vi "EC_Load.vi"() -> ()   [LabVIEW 2018]
uses:
  <vilib>/Utility/miscctls.llb/LVPositionTypeDef.ctl
panel:
  in  "Tab Control":enum32{"Document", "File"}(tab)
  in  "Document Path":path
  in  "Undo":bool
  in  "Document Tree":string[](tree)=["D:\\ATI_MS_InstrumentControl_08_08_15\\MSData\\Test\\Untitled.flist"]
  in  "File Tree":string[](tree)
  out "Navigate Tree:Get Path":string[](array[string])
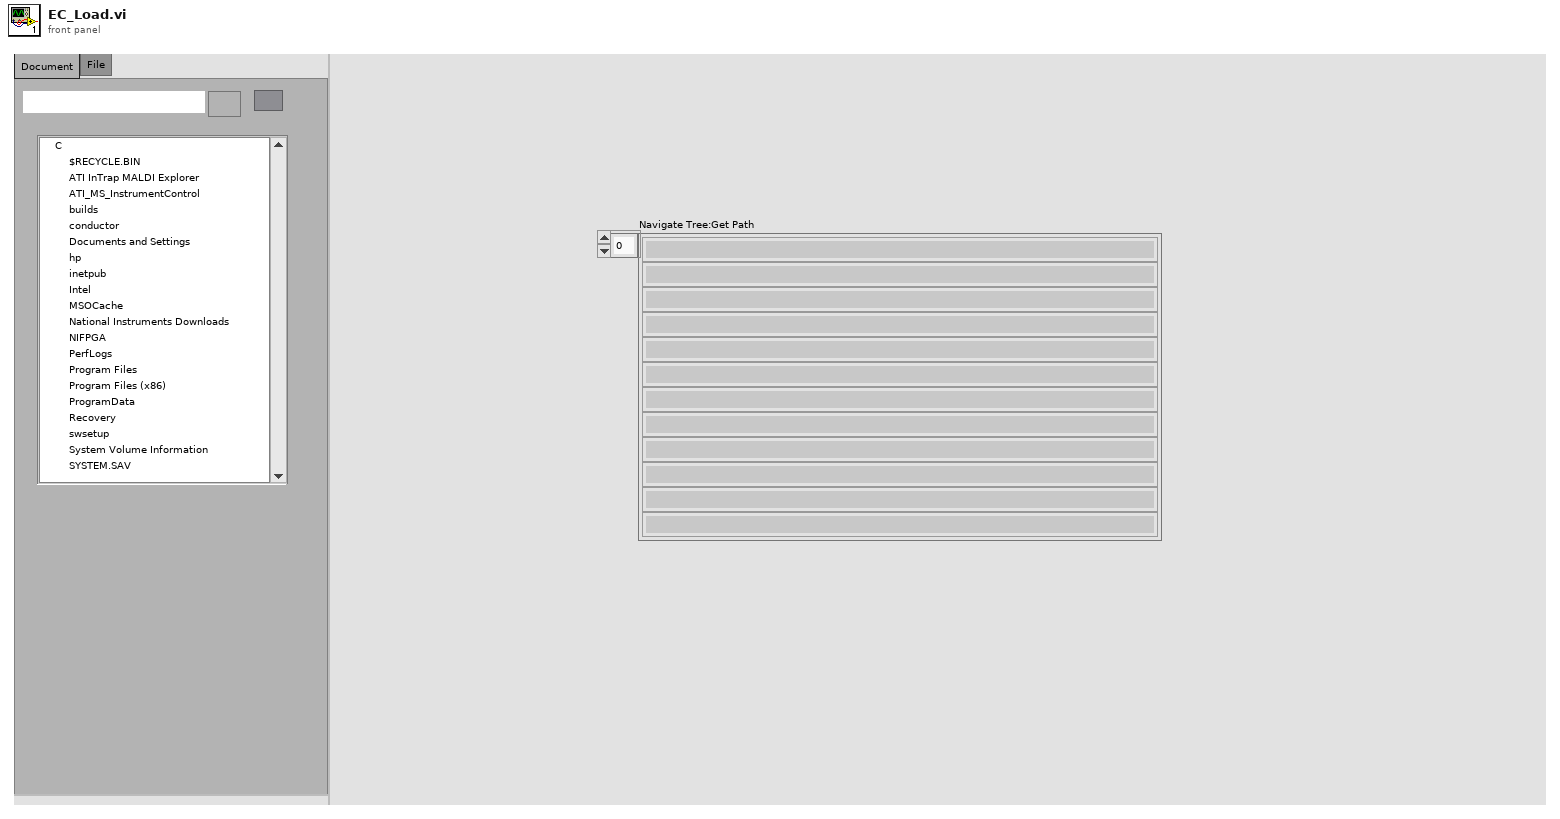
[diagram p1: front panel]
types:
  T1 = typedef "LVPositionTypeDef.ctl" = cluster{"Left":i32, "Top":i32}
  T2 = typedef "LVBoundsTypeDef.ctl" = cluster{"Width":u32, "Height":u32}
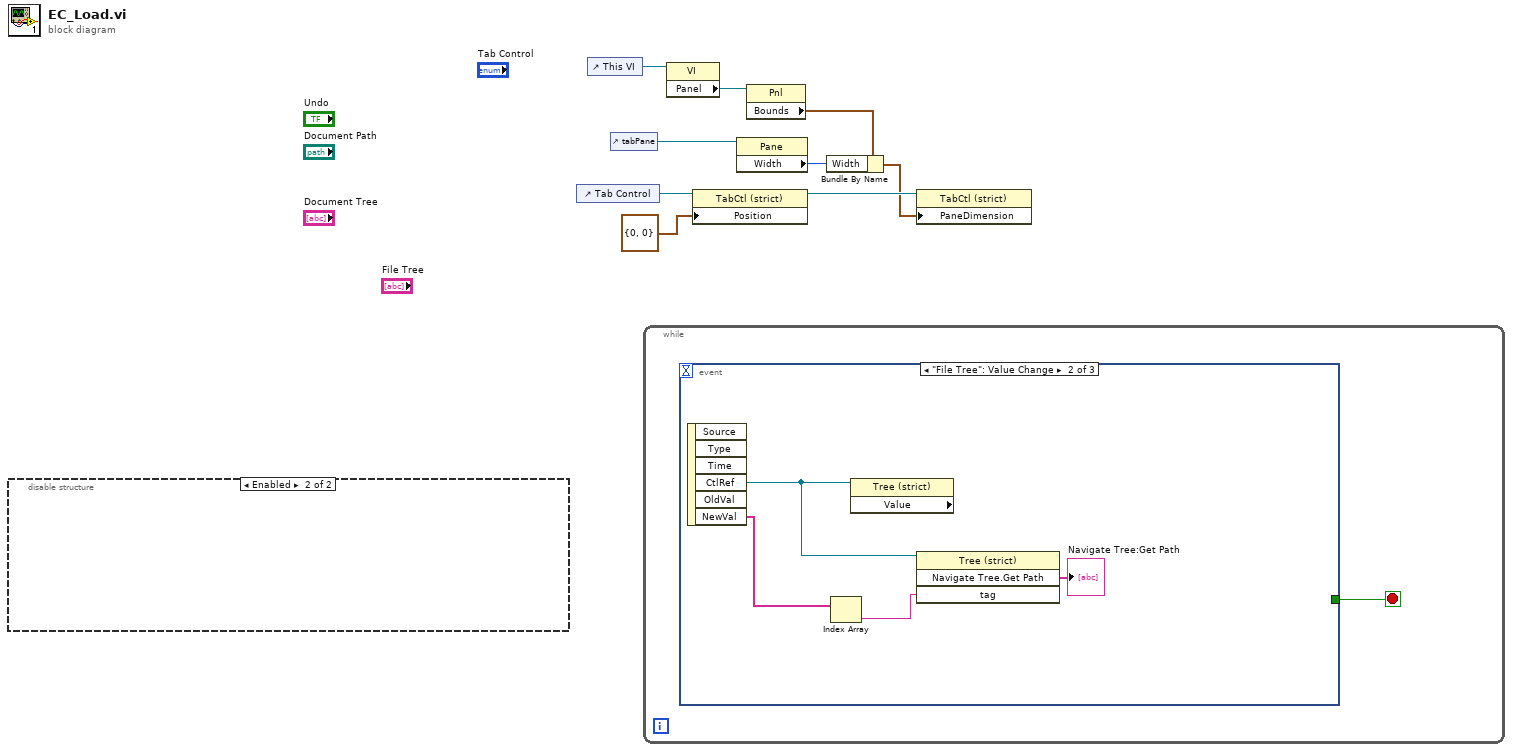
[diagram p0: block diagram]
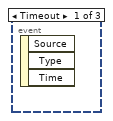
[diagram p2: hidden frame]
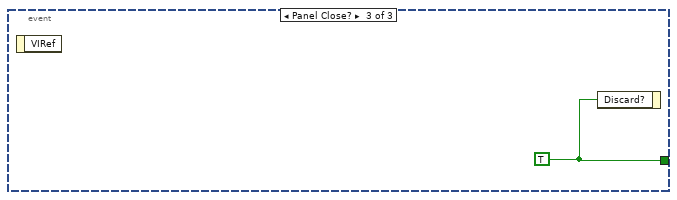
[diagram p3: hidden frame]
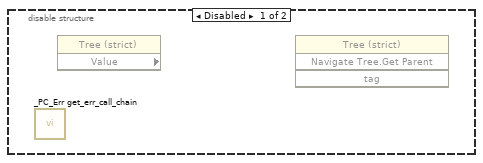
[diagram p4: hidden frame]
diagram:
  n1 = disable-structure shown="Enabled" {
    frame Disabled {
      n2 = call "_PC_Err get_err_call_chain.vi"() -> ()  [unwired: 1 out]
      n3 = property class="Tree (strict)"() -> (reference=w16:refnum<vi>, reference out=w15:refnum<vi>, error out=w14:errorcluster, "Value"=w13:string[])  [unwired: 1 in]
      n4 = invoke class="Tree (strict)" method="Navigate Tree.Get Parent"() -> (reference=w12:refnum<vi>, error in=w11:errorcluster, "tag"=w10:string)  [unwired: 1 in, 4 out]
    }
    frame Enabled {
    }
  }
  n5 = control-ref of="Tab Control"() -> (w9:refnum<vi>)
  n6 = control-ref of="This VI"() -> (w7:refnum<vi>)
  n7 = control-ref of="tabPane"() -> (w2:refnum<vi>)
  n8 = while {
    stop <- w17 stop-if-true
    n9 = event shown="[1] \"File Tree\": Value Change" {
      selector: _ -> [_ _ _]
      dyn-events: _ -> [_ _ _]
      timeout: _ -> [_ _ _]
      tunnel: [_ _ w22] -> w17
      event Timeout {
        n10 = event-data() -> ()  [unwired: 1 in, 3 out]
      }
      event "File Tree": Value Change {
        n11 = event-data() -> ("CtlRef"=w21:refnum<vi>, "NewVal"=w20:string[])  [unwired: 1 in, 4 out]
        n12 = Index Array(array=w20) -> (element=w19:string)  [unwired: 1 in]
        n13 = property class="Tree (strict)" props=["Value"](reference=w21) -> ()  [unwired: 1 in, 3 out]
        n14 = invoke class="Tree (strict)" method="Navigate Tree.Get Path"(reference=w21, "tag"=w19) -> ("Navigate Tree:Get Path"=→"Navigate Tree:Get Path":string[])  [unwired: 2 in, 3 out]
      }
      event Panel Close? {
        w22 = TRUE
        n15 = event-data() -> ()  [unwired: 1 in, 1 out]
        n16 = event-data("Discard?"=w22) -> ()  [unwired: 1 in, 1 out]
      }
    }
  }
  n17 = property class="VI"(reference=w7) -> ("Panel"=w6:refnum<vi>)  [unwired: 1 in, 2 out]
  n18 = property class="TabCtl (strict)"(reference=w9, "Position"=T1 {"Left"=0, "Top"=0}) -> (reference out=w5:refnum<vi>)  [unwired: 1 in, 1 out]
  n19 = property class="Pane"(reference=w2) -> ("Width"=w3:u32)  [unwired: 1 in, 2 out]
  n20 = property class="Pnl"(reference=w6) -> ("Bounds"=w4:T2)  [unwired: 1 in, 2 out]
  n21 = Bundle By Name(cluster=w4, "Width"=w3) -> (w1:T2)
  n22 = property class="TabCtl (strict)"(reference=w5, "PaneDimension"=w1) -> ()  [unwired: 1 in, 2 out]
